vi "explore_events4.vi"() -> ()   [LabVIEW 2023]
uses:
  <extravilib>/ChannelInstances/Event Messenger-i32.lvlib
panel:
  out "cnt":i32
  out "So error":errorcluster
  out "SO return":i32
  out "EventNR":string
  out "Numeric 2":i32
  out "error out 2":errorcluster
  out "return type":i32
  out "*(type *) &x":i32
  out "error out":errorcluster
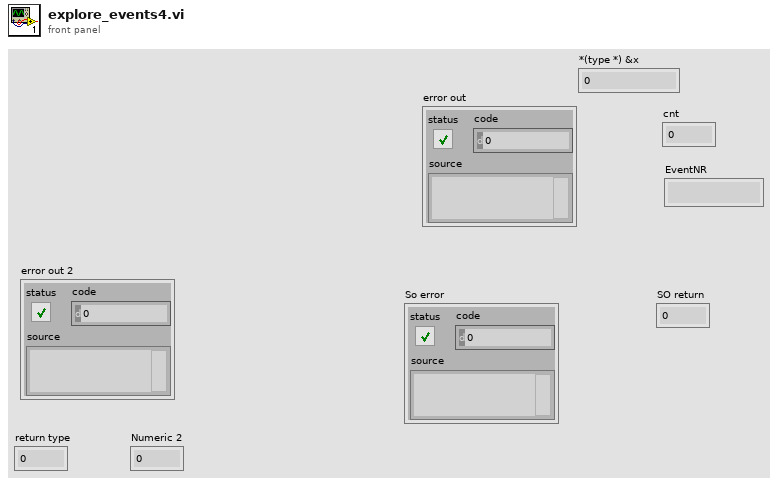
[diagram p1: front panel]
types:
  T1 = typedef "Event Messenger-i32.lvlib/))Channel.ctl" = refnum<queue>
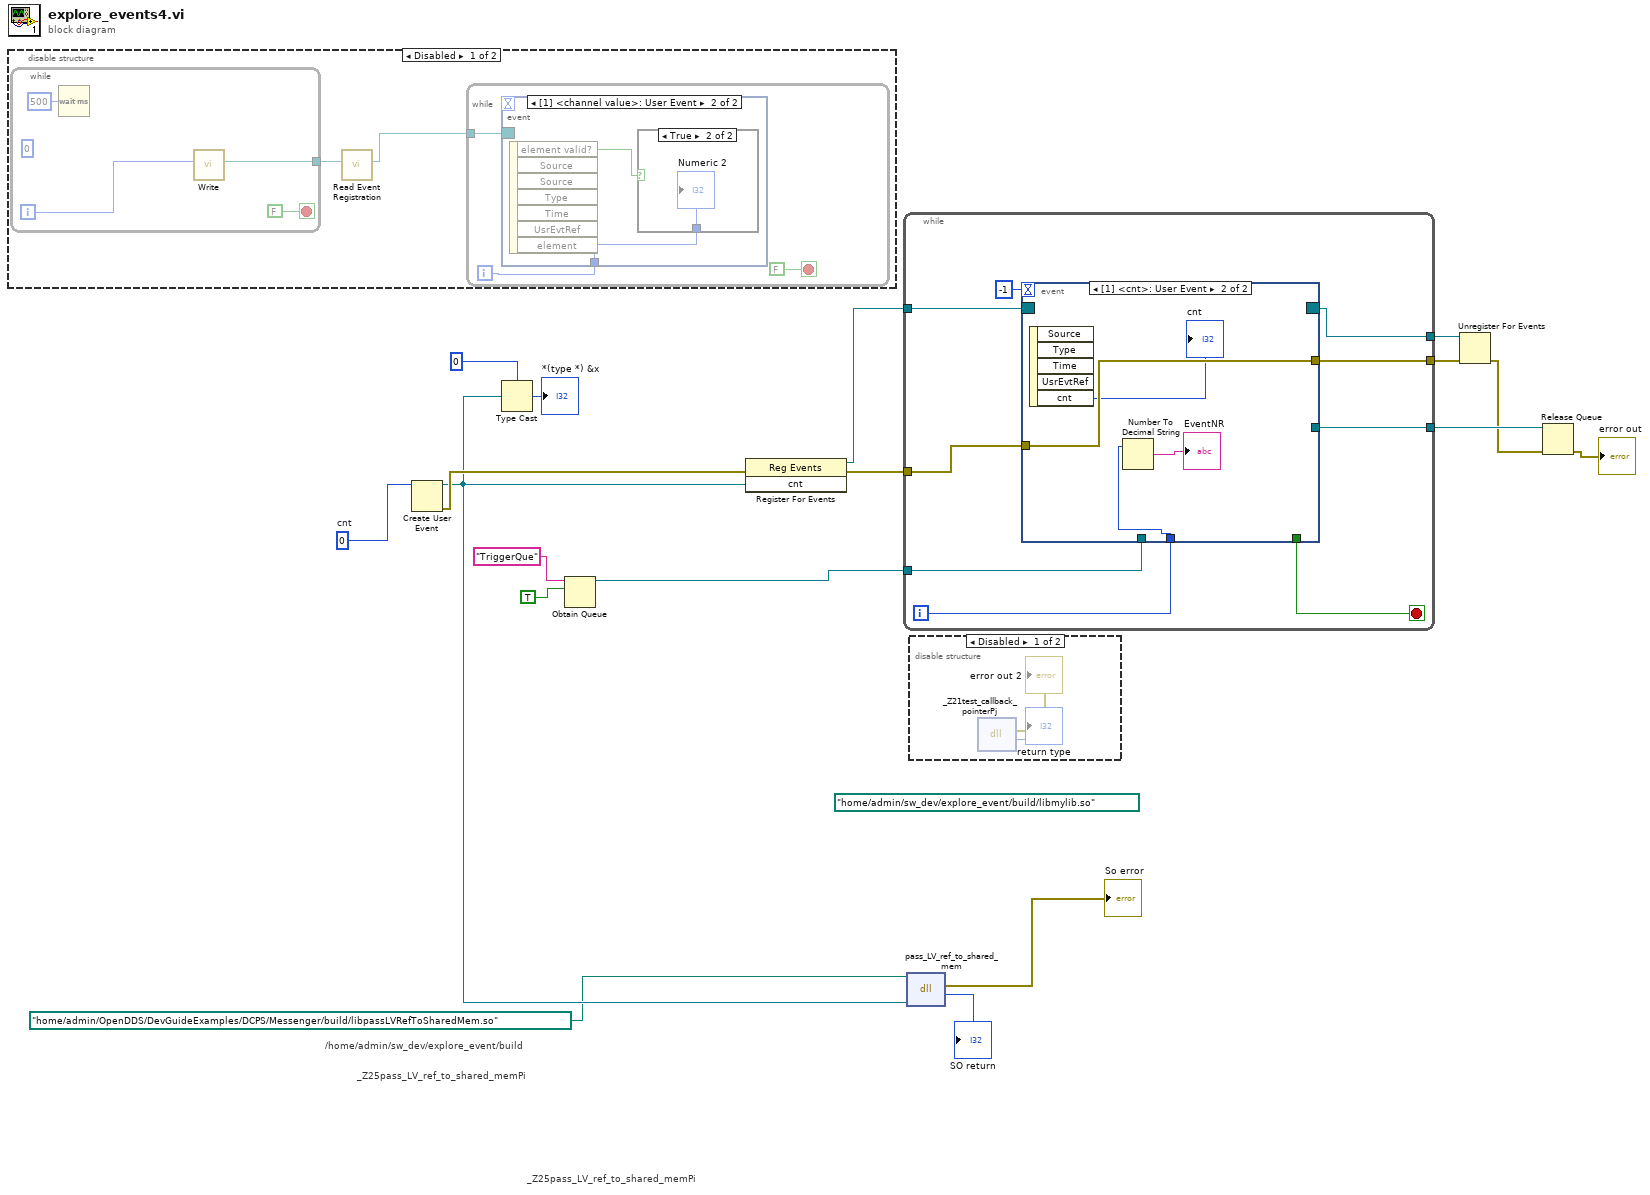
[diagram p0: block diagram]
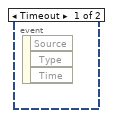
[diagram p3: hidden frame]
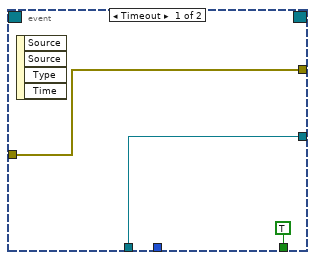
[diagram p6: hidden frame]
diagram:
  (unwired) path "/home/admin/sw_dev/explore_event/build/libmylib.so" ("path in")
  w17 = 0  # cnt
  # "_Z25pass_LV_ref_to_shared_memPi"
  # "_Z25pass_LV_ref_to_shared_memPi"
  # "/home/admin/sw_dev/explore_event/build"
  n1 = disable-structure shown="Disabled" {
    frame Disabled {
      n2 = while {
        tunnel: [w27] -> w20
        i -> [w28]
        stop <- FALSE stop-if-true
        (unwired) 0
        n3 = Wait (ms)(milliseconds to wait=u32 500) -> ()  [unwired: 1 out]
        n4 = call <extravilib>:"Write.vi"("element"=w28) -> ("channel"=w27:T1)  [unwired: 9 in, 1 out]
      }
      n5 = call <extravilib>:"Read Event Registration.vi"("channel"=w20) -> ("event registration refnum"=w19:refnum<event-registration>)  [unwired: 10 in]
      n6 = while {
        tunnel: w19 -> [w21]
        i -> [w22]
        stop <- FALSE stop-if-true
        n7 = event shown="[1] <channel value>: User Event" {
          selector: w21 -> [_ _]
          dyn-events: _ -> [_ _]
          timeout: _ -> [_ _]
          tunnel: w22 -> [_ w25]
          event Timeout {
            n8 = event-data() -> ()  [unwired: 1 in, 3 out]
          }
          event User Event {
            n9 = event-data() -> ("element valid?"=w24:bool)  [unwired: 1 in, 6 out]
            n10 = case shown="True" w24 {
              tunnel: w25 -> [_ w26]
              frame False {
              }
              frame True {
                "Numeric 2" <- w26
              }
            }
          }
        }
      }
    }
    frame Enabled {
    }
  }
  n11 = Create User Event(user event datatype=w17) -> (user event=w4:refnum<user-event>, error out=w6:errorcluster)  [unwired: 1 in]
  n12 = Type Cast(type=0, x=w4) -> (*(type *) &x=→"*(type *) &x":i32)
  n13 = Obtain Queue(name (unnamed)="TriggerQue", element data type=TRUE) -> (queue out=w13:refnum<queue>)  [unwired: 3 in, 2 out]
  n14 = register-events(error in=w6, w4) -> (reference out=w5:refnum<event-registration>, error out=w12:errorcluster)  [unwired: 1 in]
  n15 = while {
    tunnel: [w39] -> w18
    tunnel: w13 -> [w37]
    tunnel: w12 -> [w36]
    tunnel: [w34] -> w11
    tunnel: [w33] -> w9
    tunnel: w5 -> [w31]
    i -> [w38]
    stop <- w32 stop-if-true
    n16 = event shown="[1] <cnt>: User Event" {
      selector: w31 -> [_ _]
      dyn-events: [_ _] -> w39
      timeout: -1 -> [_ _]
      tunnel: w38 -> [_ w45]
      tunnel: w37 -> [w42 _]
      tunnel: w36 -> [w41 w44]
      tunnel: [w42 _] -> w34
      tunnel: [w41 w44] -> w33
      tunnel: [TRUE _] -> w32
      event Timeout {
        n17 = event-data() -> ()  [unwired: 1 in, 4 out]
      }
      event User Event {
        n18 = event-data() -> ("cnt"=→"cnt":i32)  [unwired: 1 in, 4 out]
        n19 = Number To Decimal String(number=w45) -> (decimal integer string=→"EventNR":string)  [unwired: 1 in]
      }
    }
  }
  n20 = dll-call lib="libpassLVRefToSharedMem.so" fn="pass_LV_ref_to_shared_mem"(path in=path "/home/admin/OpenDDS/DevGuideExamples/DCPS/Messenger/build/libpassLVRefToSharedMem.so", "ref"=w4) -> (error out=→"So error":errorcluster, "return type"=→"SO return":i32)  [unwired: 3 in, 1 out]
  n21 = disable-structure shown="Disabled" {
    frame Disabled {
      n22 = dll-call lib="libmylib.so" fn="_Z21test_callback_pointerPj"() -> (error out=→"error out 2":errorcluster, "return type"=→"return type":i32)  [unwired: 5 in, 1 out]
    }
    frame Enabled {
    }
  }
  n23 = Unregister For Events(event registration refnum=w18, error in=w9) -> (error out=w8:errorcluster)
  n24 = Release Queue(queue=w11, error in (no error)=w8) -> (error out=→"error out":errorcluster)  [unwired: 1 in, 2 out]
